vi "TransGenerate.vi"() -> ()   [LabVIEW 2017]
uses:
  <vilib>/Analysis/NI_AALBase.lvlib
panel:
  in  "Noise":bool
  out "Waveform Graph 3":dbl[](graph)
  in  "A1":dbl step=100.0
  in  "A2":dbl step=100.0
  in  "tau2":dbl step=0.1
  in  "t0":dbl step=0.1
  in  "tau1":dbl step=0.1
  in  "Z":dbl
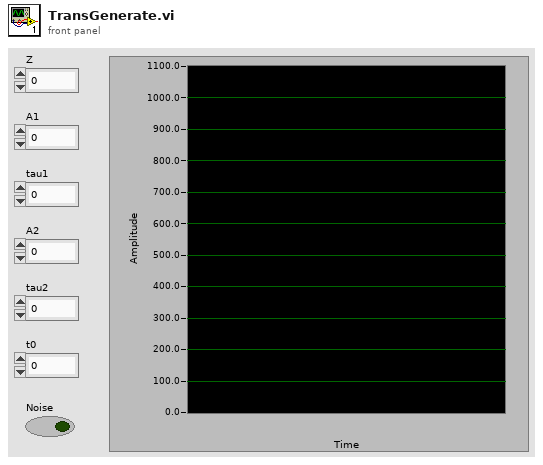
[diagram p1: front panel]
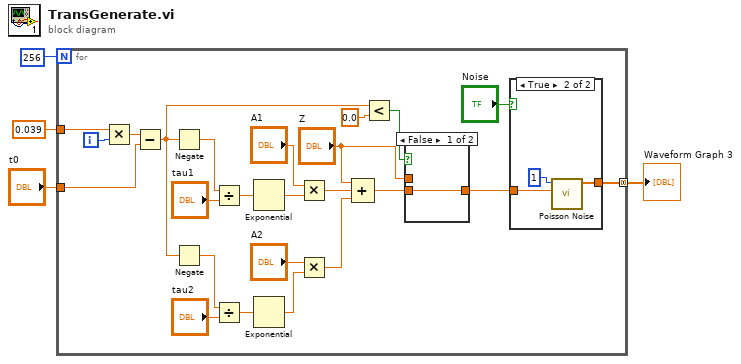
[diagram p0: block diagram]
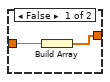
[diagram p2: hidden frame]
diagram:
  n1 = for {
    N: 256 -> [_]
    tunnel: 0.039 ("x") -> [w25]
    tunnel: "t0" -> [w13]
    tunnel: [w8] -> w2 mode=concatenating
    i -> [w6]
    n2 = Multiply(x=w25, y=w6) -> (x*y=w12:dbl)
    n3 = Subtract(x=w12, y=w13) -> (x-y=w5:dbl)
    n4 = Negate(x=w5) -> (-x=w26:dbl)
    n5 = Negate(x=w5) -> (-x=w22:dbl)
    n6 = Divide(x=w26, y="tau1") -> (x/y=w28:dbl)
    n7 = Divide(x=w22, y="tau2") -> (x/y=w21:dbl)
    n8 = Exponential(1:w28) -> (0:w15:dbl)
    n9 = Exponential(1:w21) -> (0:w19:dbl)
    n10 = Multiply(x="A1", y=w15) -> (x*y=w16:dbl)
    n11 = Multiply(x="A2", y=w19) -> (x*y=w18:dbl)
    n12 = Compound Arithmetic op=ADD("Z", w16, w18) -> (w20:dbl)
    n13 = Less?(x=w5, y=0.0) -> (x < y?=w24:bool)
    n14 = case shown="False" w24 {
      tunnel: [w34 w35] -> w9
      tunnel: w20 -> [w34 _]
      tunnel: "Z" -> [_ w35]
      frame False {
      }
      frame True {
      }
    }
    n15 = case shown="True" "Noise" {
      tunnel: w9 -> [w30 w31]
      tunnel: [w29 w32] -> w8
      frame False {
        n16 = Build Array(w30) -> (w29:dbl[])
      }
      frame True {
        n17 = call <vilib>:"Poisson Noise.vi"("mean"=w31, "samples"=1) -> ("poisson noise"=w32:dbl[])  [unwired: 8 in, 1 out]
      }
    }
  }
  "Waveform Graph 3" <- w2
